vi "PumpValveHeater3.vi"() -> ()   [LabVIEW 2015]
uses:
  PumpValve.ctl
  <vilib>/DAQmx/read.llb/DAQmx Read (Analog 1D Wfm NChan 1Samp).vi
  <vilib>/DAQmx/write.llb/DAQmx Write (Digital 1D Bool NChan 1Samp 1Line).vi
  <vilib>/DAQmx/miscellaneous.llb/DAQmx Fill In Error Info.vi
  <vilib>/addons/control/pid/pid.llb/PID Advanced (DBL).vi
  <vilib>/addons/control/pid/NI_PID_pid.lvlib
panel:
  out "Pressure (mBar)":dbl format="%#_13g"
  out "Voltage Reading (Pressure)":dbl format="%#_13g"
  out "Pressure Chart Voltage":waveform(dbl)(graph)
  out "Voltage Reading(Temp)":dbl format="%#_13g"
  out "Temperature (Celcius)":dbl format="%#_13g"
  out "Temp(C)":dbl(slide) scale=-10.0..100.0
  out "Temp Chart":waveform(dbl)(graph)
  out "Duty Cycle from Control Value":dbl
  out "Control Value Pressure":dbl
  out "Heater On/off":bool
  out "Control Value (Temp Sensor)":dbl(knob) scale=0.0..100.0
  in  "PID gains Temp":T1={"proportional gain (Kc)"=1.0, "integral time (Ti, min)"=0.01, "derivative time (Td, min)"=0.0} {"derivative time (Td, min)" format="%.3f"; "integral time (Ti, min)" format="%.3f"; "proportional gain (Kc)" format="%.3f"}
  in  "Temp Setting":dbl
  in  "Maintain Temp":bool
  in  "Stop Maintaining Pressure":bool
  in  "PID gains":T1={"proportional gain (Kc)"=1.0, "integral time (Ti, min)"=0.01, "derivative time (Td, min)"=0.0} {"derivative time (Td, min)" format="%.3f"; "integral time (Ti, min)" format="%.3f"; "proportional gain (Kc)" format="%.3f"}
  out "Control Value (Pressure Sensor)":dbl(knob) scale=-10.0..10.0
  in  "Pressure Setting (mBar)":dbl
  in  "Maintain pressure":bool
  in  "On/Off Temp":bool
  in  "Manual Mode Temp":bool
  in  "Duty cycle % (0-100)":dbl=50.0
  in  "Steps in a cycle":i32=256
  in  "Cycle time (s)":dbl=5.0
  in  "On/Off (Pump)":bool
  in  "Open/Close (Blue)":bool
  in  "Open/Close (Green)":bool
  in  "Manual Mode Pump/Valve":bool
  out "Invalid fill%":bool
  out "Tank":u32(slide) scale=0.0..100.0
  in  "Drain %":u32
  in  "Fill %":u32
  in  "Drain":bool
  in  "Stop Program":bool
  in  "Fill":bool
  # "Temp only adjusts up (do nothing to cool?)"
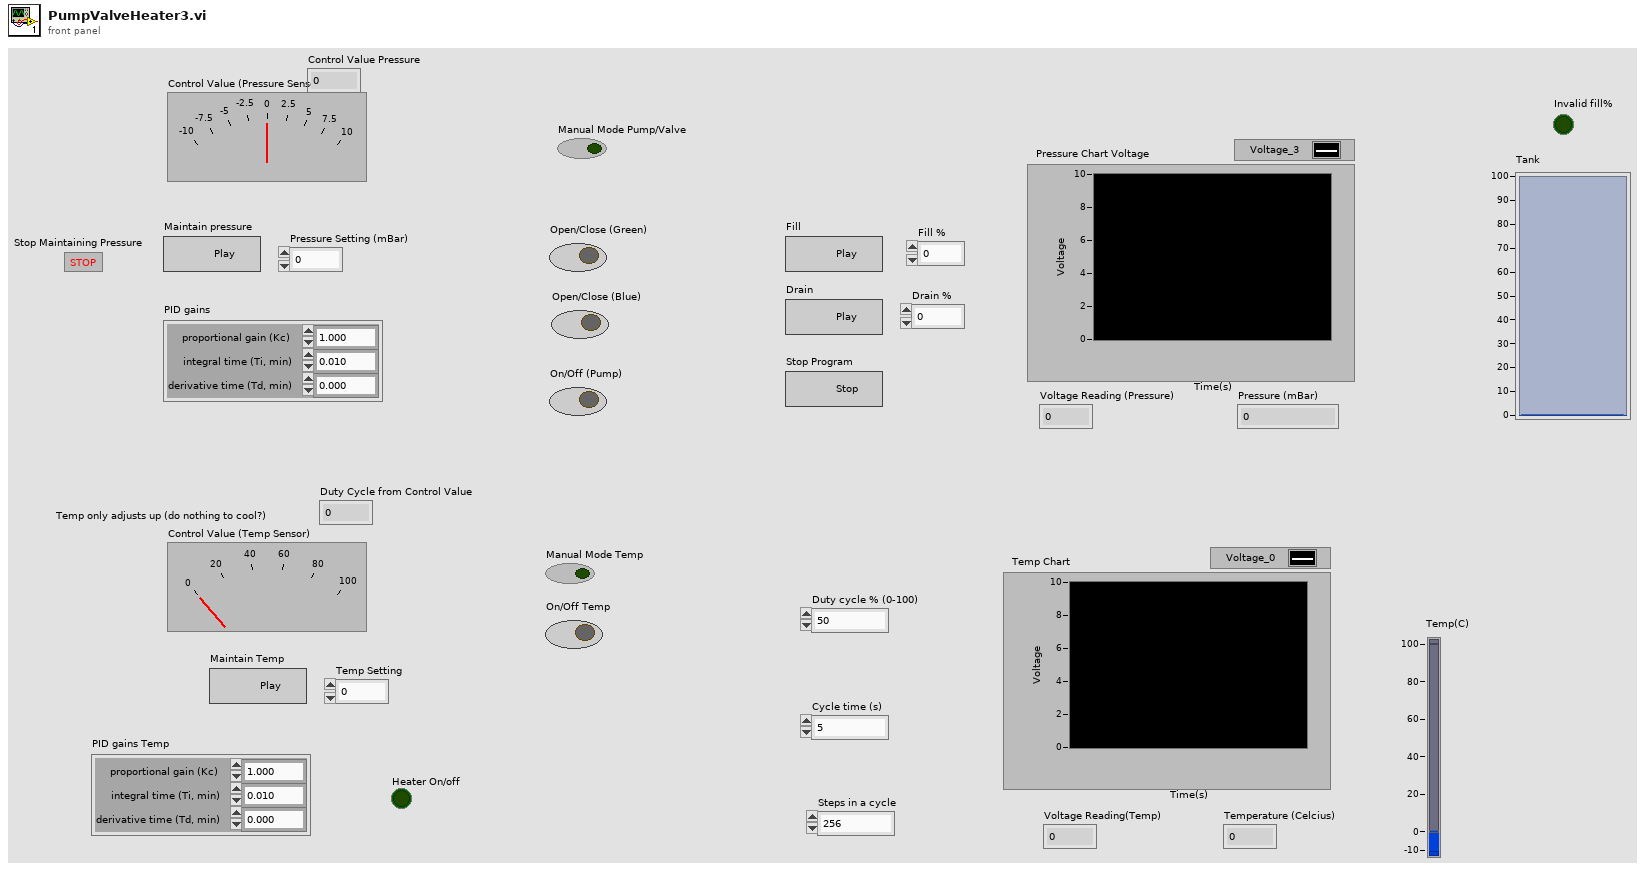
[diagram p1: front panel]
types:
  T1 = cluster{"proportional gain (Kc)":dbl, "integral time (Ti, min)":dbl, "derivative time (Td, min)":dbl}
  T2 = typedef "PumpValve.ctl" = enum16{"PressureSetting", "ManualPressure", "ManualTemp", "Idle Temp", "Set Temp", "Initialize", "Idle", "Fill", "Drain", "Stop"}
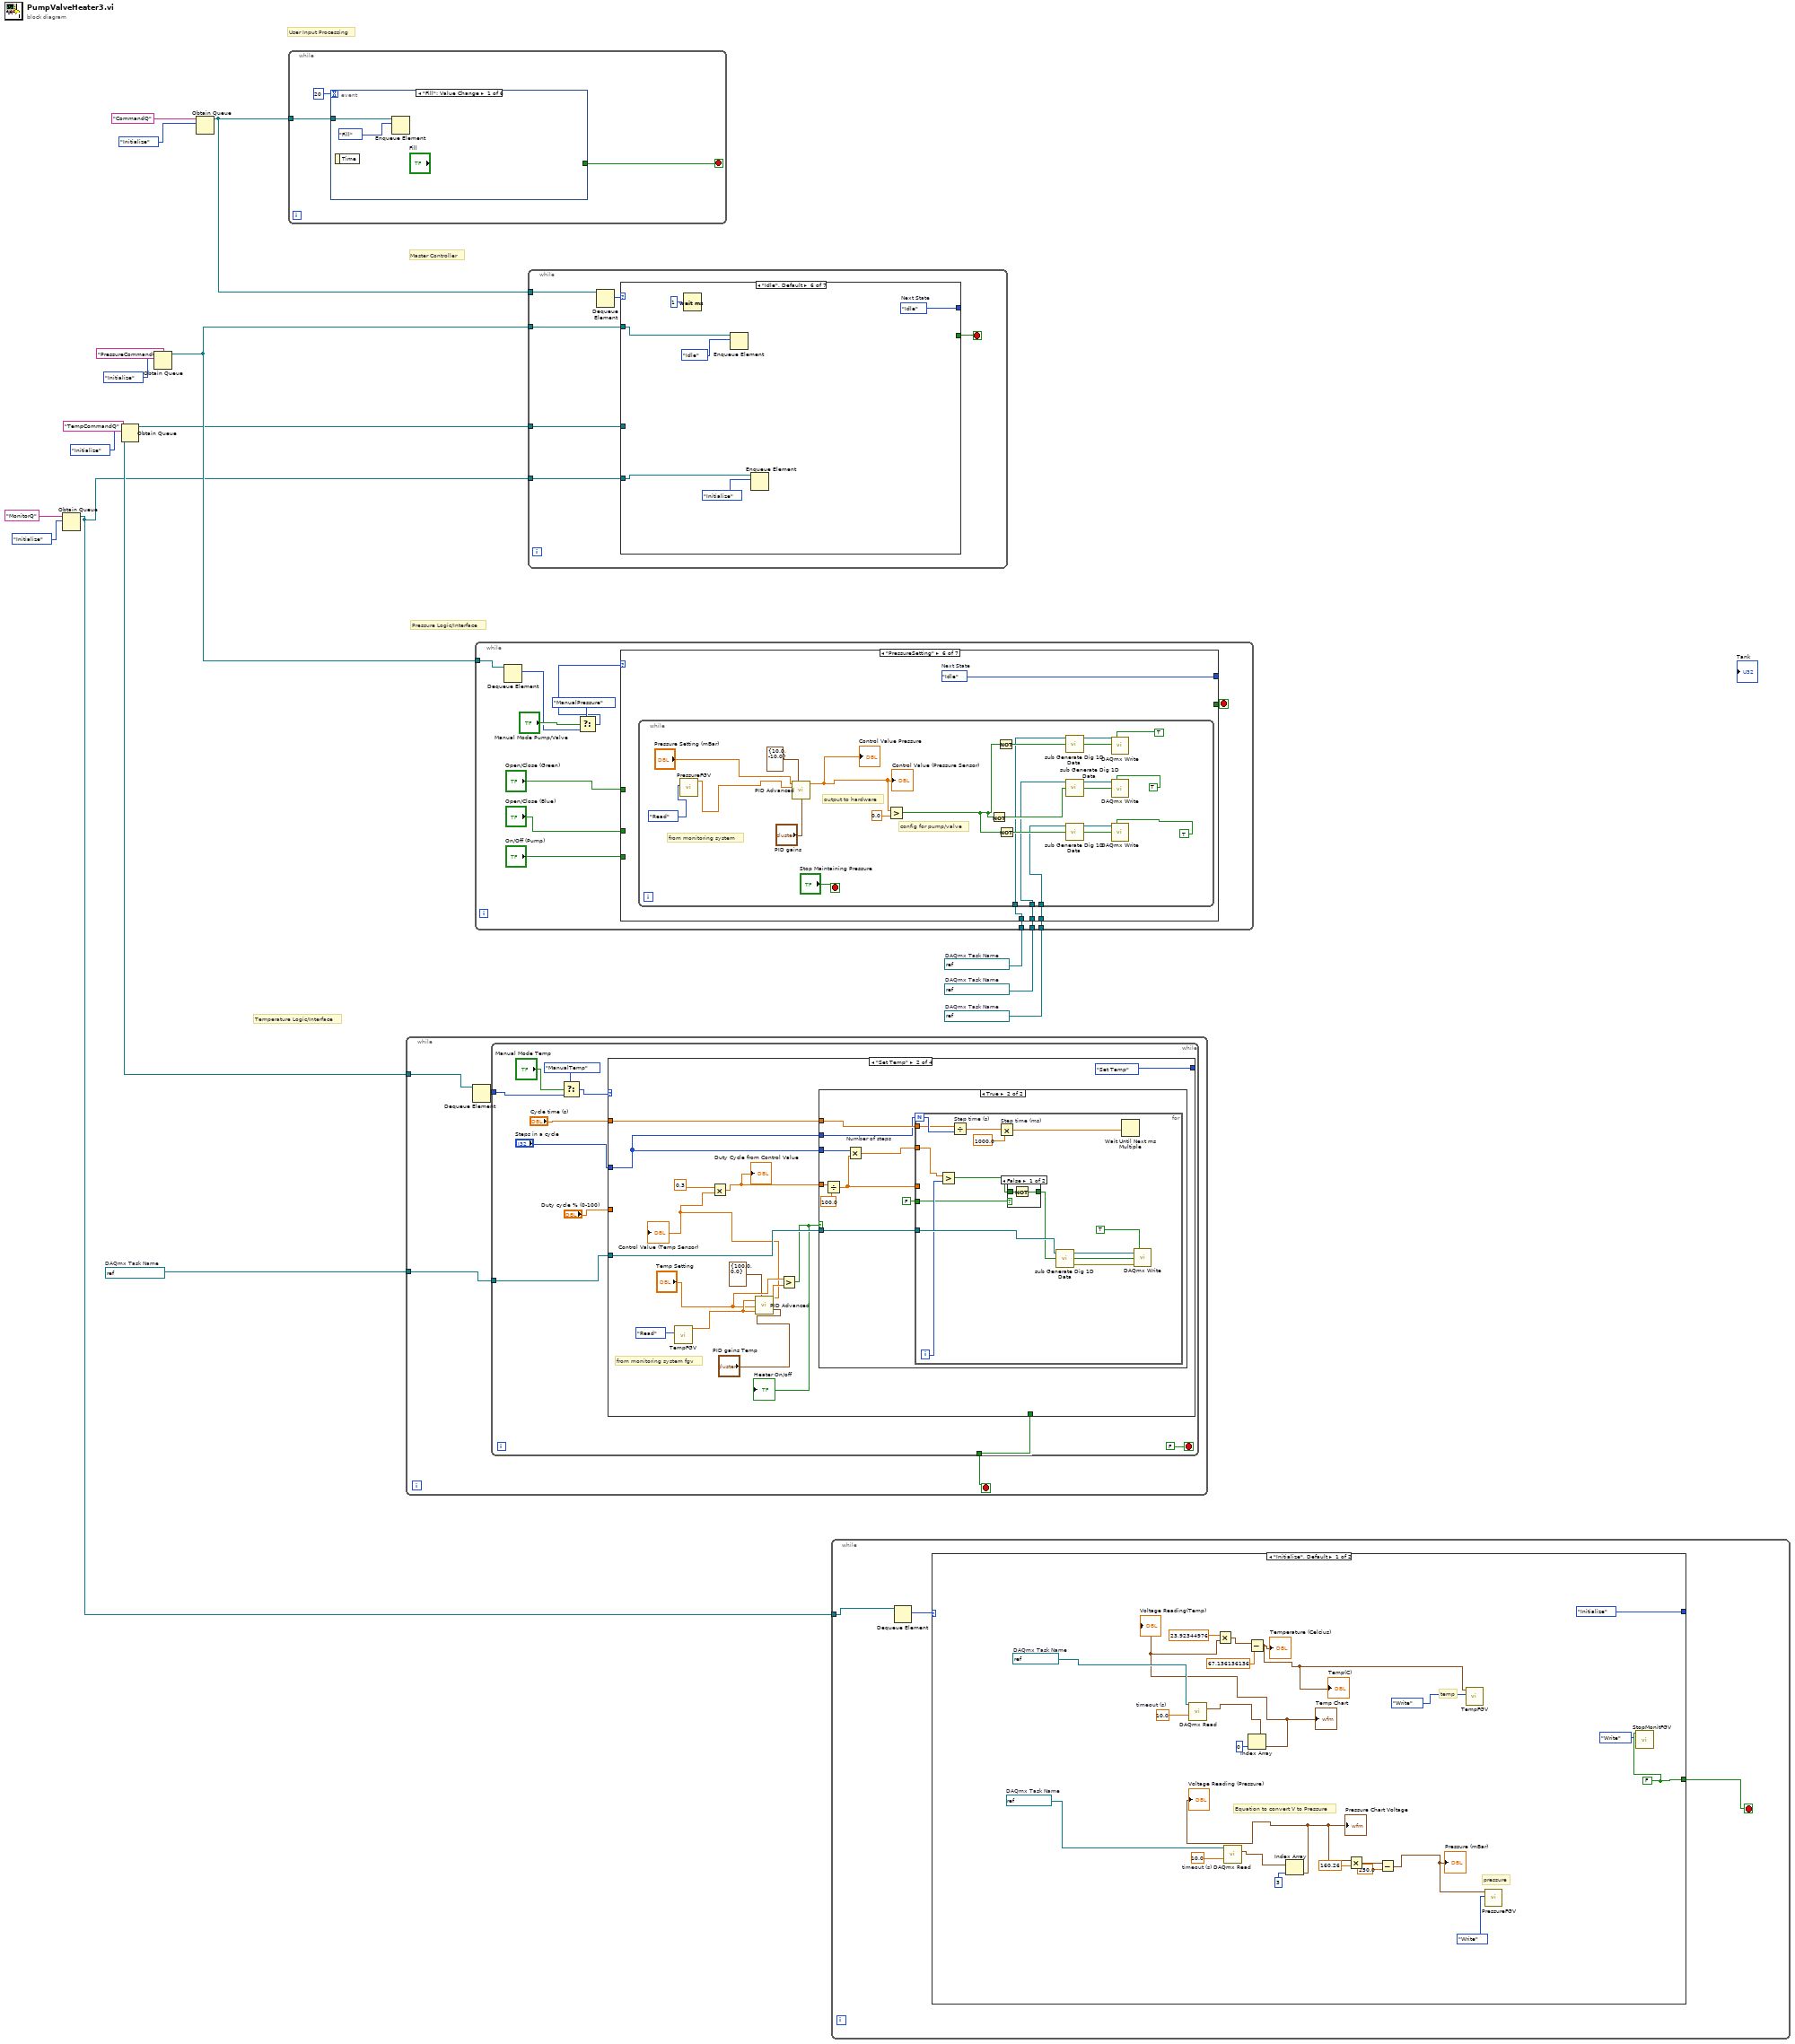
[diagram p0: block diagram]
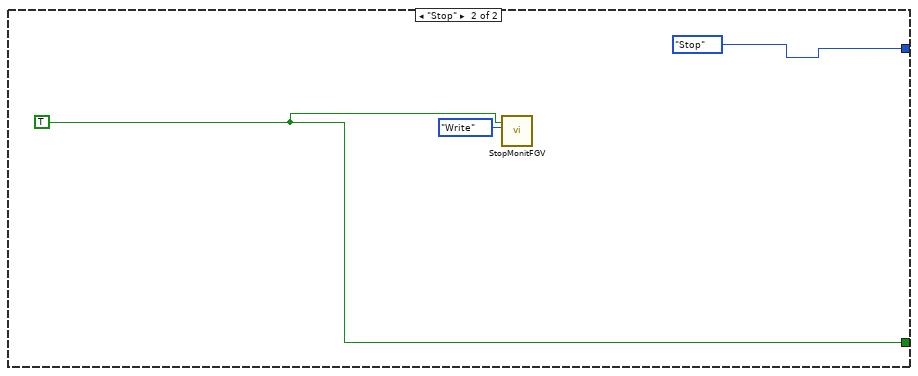
[diagram p2: hidden frame]
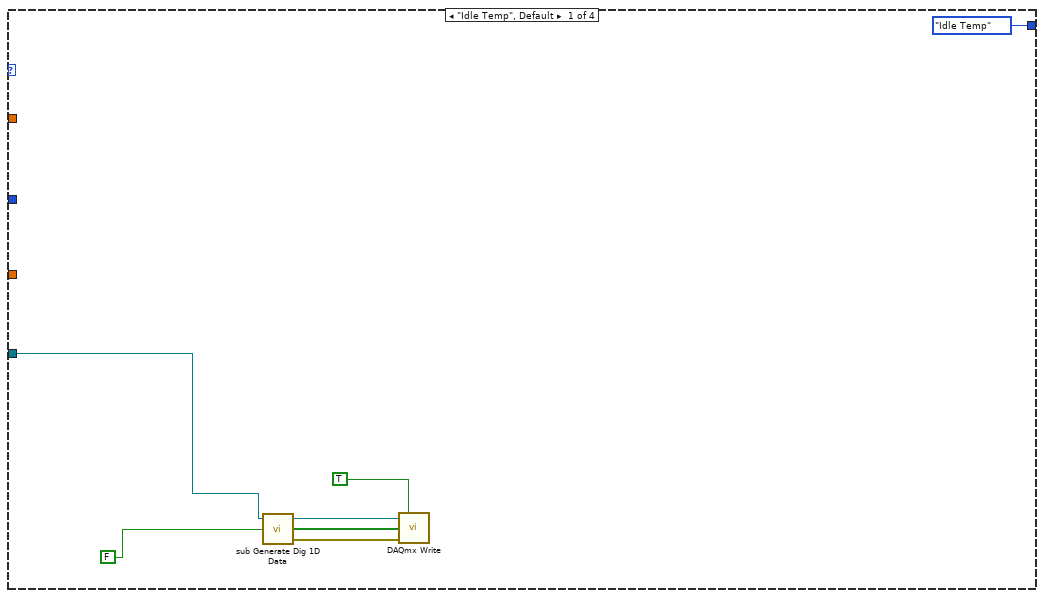
[diagram p3: hidden frame]
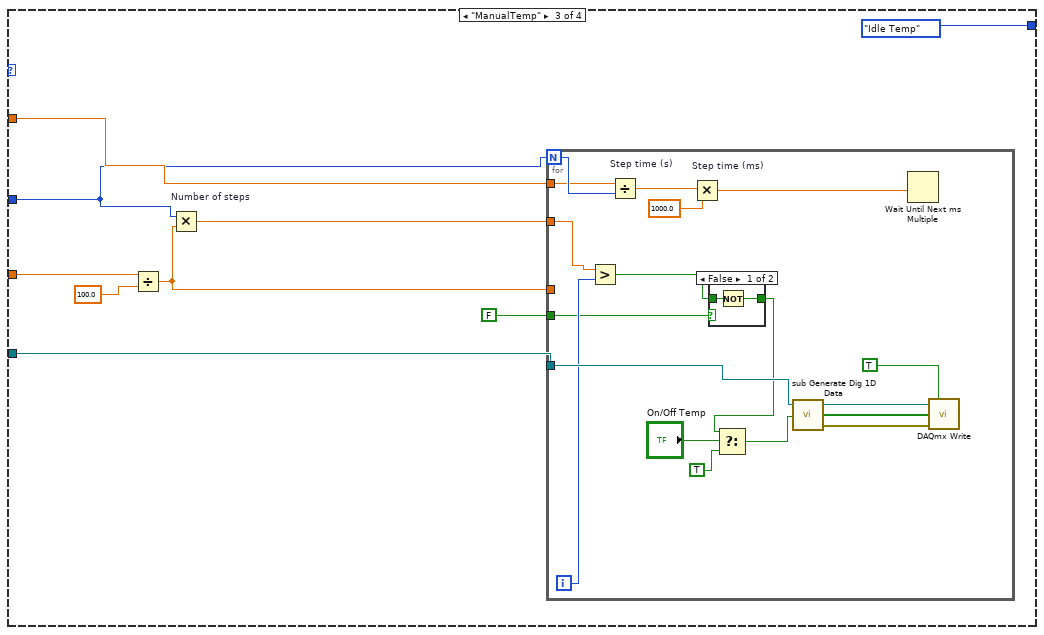
[diagram p6: hidden frame]
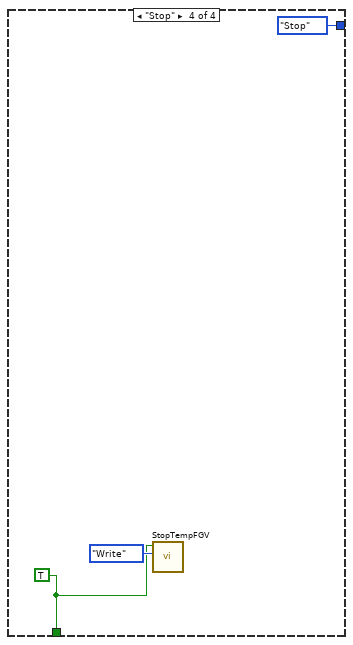
[diagram p8: hidden frame]
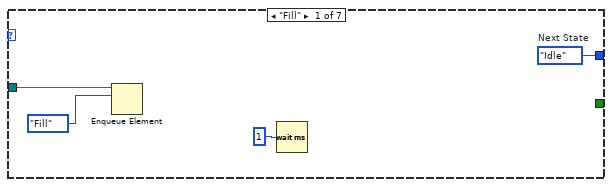
[diagram p9: hidden frame]
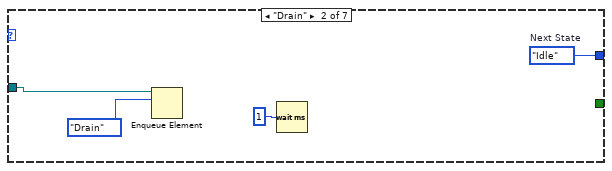
[diagram p10: hidden frame]
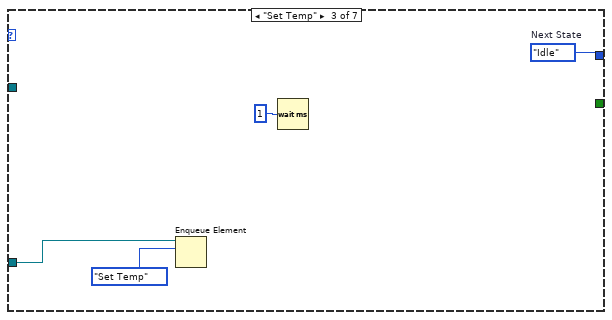
[diagram p11: hidden frame]
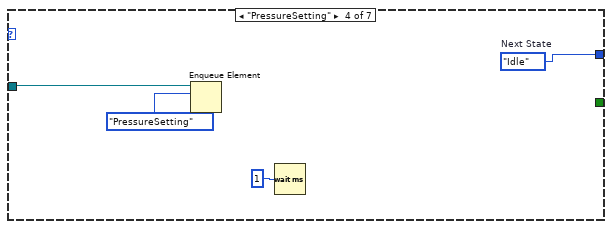
[diagram p12: hidden frame]
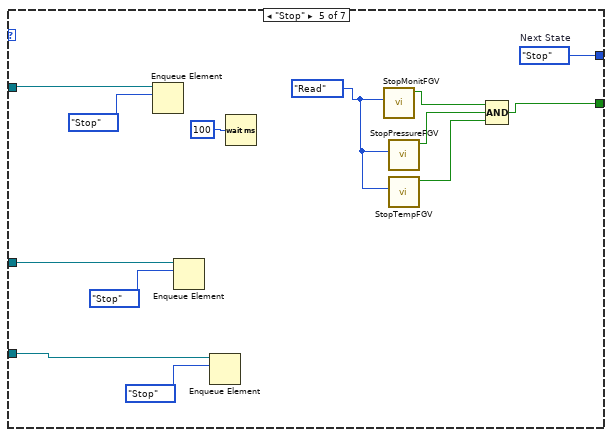
[diagram p13: hidden frame]
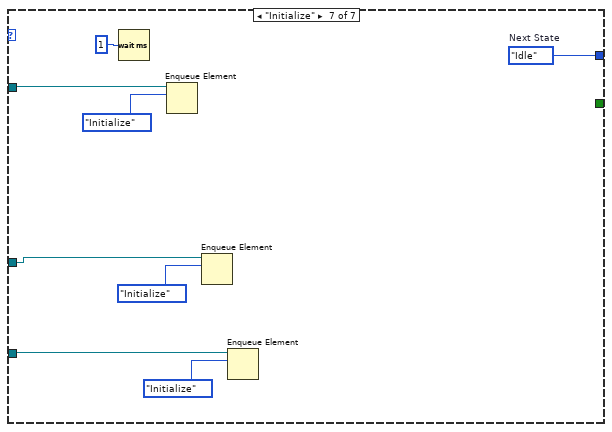
[diagram p14: hidden frame]
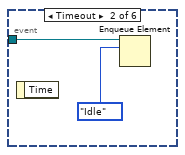
[diagram p15: hidden frame]
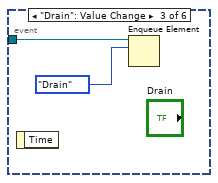
[diagram p16: hidden frame]
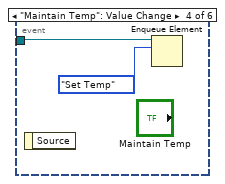
[diagram p17: hidden frame]
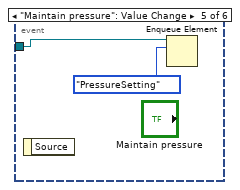
[diagram p18: hidden frame]
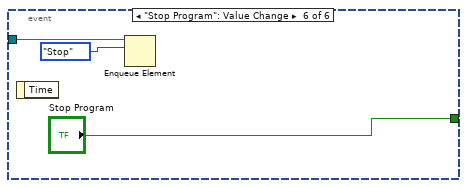
[diagram p19: hidden frame]
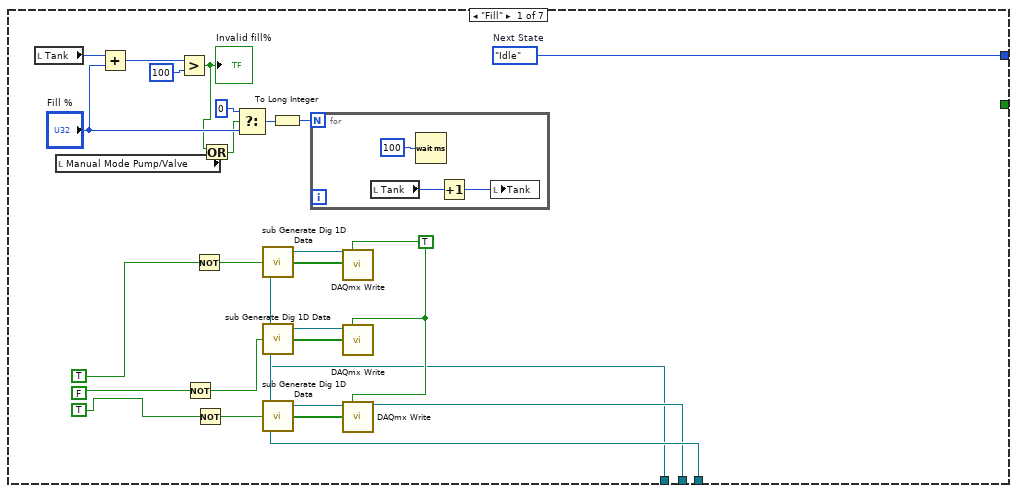
[diagram p20: hidden frame]
diagram:
  w7 = refnum<k21> "YellowdigOUT"  # DAQmx Task Name
  w12 = refnum<k21> "DigitalOutGreen"  # DAQmx Task Name
  w13 = refnum<k21> "DigitalOutGreen"  # DAQmx Task Name
  w14 = refnum<k21> "DigitalOutGreen"  # DAQmx Task Name
  # "Temperature Logic/Interface"
  # "Pressure Logic/Interface"
  # "Master Controller"
  # "User Input Processing"
  n1 = Obtain Queue(name (unnamed)="MonitorQ", element data type=PumpValve."Initialize" ("States")) -> (queue out=w1:refnum<queue>)  [unwired: 3 in, 2 out]
  n2 = Obtain Queue(name (unnamed)="TempCommandQ", element data type=PumpValve."Initialize" ("States")) -> (queue out=w4:refnum<queue>)  [unwired: 3 in, 2 out]
  n3 = Obtain Queue(name (unnamed)="PressureCommandQ", element data type=PumpValve."Initialize" ("States")) -> (queue out=w8:refnum<queue>)  [unwired: 3 in, 2 out]
  n4 = Obtain Queue(name (unnamed)="CommandQ", element data type=PumpValve."Initialize" ("States")) -> (queue out=w11:refnum<queue>)  [unwired: 3 in, 2 out]
  n5 = while {
    tunnel: w11 -> [w18]
    stop <- w17 stop-if-true
    n6 = event shown="[0] \"Fill\": Value Change" {
      selector: _ -> [_ _ _ _ _ _]
      dyn-events: _ -> [_ _ _ _ _ _]
      timeout: 20 -> [_ _ _ _ _ _]
      tunnel: w18 -> [w21 w23 w25 w26 w29 w32]
      tunnel: [_ _ _ _ _ "Stop Program"] -> w17
      event "Fill": Value Change {
        n7 = event-data() -> ()  [unwired: 1 in, 1 out]
        n8 = Enqueue Element(queue=w21, element=PumpValve."Fill" ("States")) -> ()  [unwired: 2 in, 3 out]
      }
      event Timeout {
        n9 = event-data() -> ()  [unwired: 1 in, 1 out]
        n10 = Enqueue Element(queue=w23, element=PumpValve."Idle" ("States")) -> ()  [unwired: 2 in, 3 out]
      }
      event "Drain": Value Change {
        n11 = event-data() -> ()  [unwired: 1 in, 1 out]
        n12 = Enqueue Element(queue=w25, element=PumpValve."Drain" ("States")) -> ()  [unwired: 2 in, 3 out]
      }
      event "Maintain Temp": Value Change {
        n13 = event-data() -> ()  [unwired: 1 in, 1 out]
        n14 = Enqueue Element(queue=w26, element=PumpValve."Set Temp" ("States")) -> ()  [unwired: 2 in, 3 out]
      }
      event "Maintain pressure": Value Change {
        n15 = event-data() -> ()  [unwired: 1 in, 1 out]
        n16 = Enqueue Element(queue=w29, element=PumpValve."PressureSetting" ("States")) -> ()  [unwired: 2 in, 3 out]
      }
      event "Stop Program": Value Change {
        n17 = event-data() -> ()  [unwired: 1 in, 1 out]
        n18 = Enqueue Element(queue=w32, element=PumpValve."Stop" ("States")) -> ()  [unwired: 2 in, 3 out]
      }
    }
  }
  n19 = while {
    tunnel: w7 -> [w36]
    tunnel: w4 -> [w35]
    stop <- w33 stop-if-true
    n20 = Dequeue Element(queue=w35) -> (element=w34:T2)  [unwired: 2 in, 3 out]
    n21 = while {
      tunnel: w36 -> [w46]
      tunnel: w34 -> [w45]
      tunnel: [w44] -> w33
      stop <- FALSE stop-if-true
      n22 = Select(t=PumpValve."ManualTemp", s="Manual Mode Temp", f=w45) -> (s? t:f=w40:T2)
      n23 = case shown="\"Set Temp\"" w40 {
        tunnel: w46 -> [w48 w66 w101 _]
        tunnel: [PumpValve."Idle Temp" ("States") PumpValve."Set Temp" ("States") PumpValve."Idle Temp" ("States") PumpValve."Stop" ("States")] -> _
        tunnel: "Cycle time (s)" -> [_ w64 w95 _]
        tunnel: "Steps in a cycle" -> [_ w63 w94 _]
        tunnel: "Duty cycle % (0-100)" -> [_ _ w93 _]
        tunnel: [_ _ _ w124] -> w44
        frame "Idle Temp", Default {
          n24 = call <vilib>:"sub Generate Dig 1D Data.vi"("initial value"=FALSE, "task in"=w48) -> ("error out"=w50:errorcluster, "Data"=w51:bool[], "task out"=w52:refnum<k21>)  [unwired: 1 in]
          n25 = call-poly <vilib>:"DAQmx Write.vi"("task/channels in"=w52, "auto start"=TRUE, "data"=w51, "error in"=w50) -> ()  [unwired: 9 in, 3 out]
        }
        frame "Set Temp" {
          # "from monitoring system fgv"
          n26 = call "TempFGV.vi"("Command"=enum16{"Write", "Read"}."Read") -> ("OUT"=w57:dbl)  [unwired: 10 in]
          n27 = call-poly <vilib>:"PID Advanced.vi"("setpoint"="Temp Setting", "output range"=cluster{"output high":dbl, "output low":dbl} {"output high"=100.0, "output low"=0.0}, "process variable"=w57, "PID gains"="PID gains Temp") -> ("output"=w55:dbl)  [unwired: 10 in, 1 out]
          "Control Value (Temp Sensor)" <- w55
          n28 = Multiply(x=0.3, y=w55) -> (x*y=w59:dbl)
          "Duty Cycle from Control Value" <- w59
          n29 = Greater?(x="Temp Setting", y=w57) -> (0:w62:bool)
          "Heater On/off" <- w62
          n30 = case shown="True" w62 {
            tunnel: w66 -> [_ w74]
            tunnel: w64 -> [_ w69]
            tunnel: w63 -> [_ w68]
            tunnel: w59 -> [_ w67]
            tunnel: w63 -> [_ _]
            frame False {
            }
            frame True {
              n31 = Divide(x=w67, y=100.0) -> (x/y=w72:dbl)
              n32 = Multiply "Number of steps"(x=w68, y=w72) -> (x*y=w71:dbl)
              n33 = for {
                N: w68 -> [w84]
                tunnel: w74 -> [w86]
                tunnel: w72 -> [_]
                tunnel: w69 -> [w83]
                tunnel: w71 -> [w79]
                tunnel: FALSE -> [w76]
                i -> [w78]
                n34 = Greater?(x=w79, y=w78) -> (0:w77:bool)
                n35 = Divide "Step time (s)"(x=w83, y=w84) -> (x/y=w82:dbl)
                n36 = Multiply "Step time (ms)"(x=w82, y=1000.0) -> (x*y=w80:dbl)
                n37 = case shown="False" w76 {
                  tunnel: [w90 w92] -> w85
                  tunnel: w77 -> [w91 w92]
                  frame False {
                    n38 = Not(x=w91) -> (.not. x?=w90:bool)
                  }
                  frame True {
                  }
                }
                n39 = call <vilib>:"sub Generate Dig 1D Data.vi"("initial value"=w85, "task in"=w86) -> ("error out"=w88:errorcluster, "Data"=w75:bool[], "task out"=w87:refnum<k21>)  [unwired: 1 in]
                n40 = Wait Until Next ms Multiple(millisecond multiple=w80) -> ()  [unwired: 1 out]
                n41 = call-poly <vilib>:"DAQmx Write.vi"("task/channels in"=w87, "auto start"=TRUE, "data"=w75, "error in"=w88) -> ()  [unwired: 9 in, 3 out]
              }
            }
          }
        }
        frame "ManualTemp" {
          n42 = Divide(x=w93, y=100.0) -> (x/y=w99:dbl)
          n43 = Multiply "Number of steps"(x=w94, y=w99) -> (x*y=w98:dbl)
          n44 = for {
            N: w94 -> [w114]
            tunnel: w101 -> [w115]
            tunnel: w99 -> [_]
            tunnel: w95 -> [w113]
            tunnel: w98 -> [w109]
            tunnel: FALSE -> [w106]
            i -> [w108]
            n45 = Greater?(x=w109, y=w108) -> (0:w107:bool)
            n46 = Divide "Step time (s)"(x=w113, y=w114) -> (x/y=w112:dbl)
            n47 = Multiply "Step time (ms)"(x=w112, y=1000.0) -> (x*y=w110:dbl)
            n48 = case shown="False" w106 {
              tunnel: [w120 w122] -> w104
              tunnel: w107 -> [w121 w122]
              frame False {
                n49 = Not(x=w121) -> (.not. x?=w120:bool)
              }
              frame True {
              }
            }
            n50 = Select(t=w104, s="On/Off Temp", f=TRUE) -> (s? t:f=w103:bool)
            n51 = call <vilib>:"sub Generate Dig 1D Data.vi"("initial value"=w103, "task in"=w115) -> ("error out"=w118:errorcluster, "Data"=w117:bool[], "task out"=w116:refnum<k21>)  [unwired: 1 in]
            n52 = Wait Until Next ms Multiple(millisecond multiple=w110) -> ()  [unwired: 1 out]
            n53 = call-poly <vilib>:"DAQmx Write.vi"("task/channels in"=w116, "auto start"=TRUE, "data"=w117, "error in"=w118) -> ()  [unwired: 9 in, 3 out]
          }
        }
        frame "Stop" {
          w124 = TRUE
          n54 = call "StopTempFGV.vi"("Command"=enum16{"Write", "Read"}."Write", "IN"=w124) -> ()  [unwired: 9 in, 1 out]
        }
      }
    }
  }
  n55 = while {
    tunnel: w8 -> [w137]
    tunnel: w14 -> [w133]
    tunnel: w13 -> [w134]
    tunnel: w12 -> [w135]
    stop <- w136 stop-if-true
    n56 = Dequeue Element(queue=w137) -> (element=w130:T2)  [unwired: 2 in, 3 out]
    n57 = Select(t=PumpValve."ManualPressure", s="Manual Mode Pump/Valve", f=w130) -> (s? t:f=w129:T2)
    n58 = case shown="\"PressureSetting\"" w129 {
      tunnel: [w164 w192 w214 w236 w256 w260 w306] -> _
      tunnel: [_ _ w197 _ _ _ _] -> w136
      tunnel: w135 -> [w146 w174 w204 w224 w244 w257 w295]
      tunnel: w134 -> [w145 w175 w205 w223 w243 w258 w296]
      tunnel: w133 -> [w144 w176 w206 w222 w242 w259 w297]
      tunnel: "Open/Close (Green)" -> [_ _ _ _ w239 _ _]
      tunnel: "Open/Close (Blue)" -> [_ _ _ _ w238 _ _]
      tunnel: "On/Off (Pump)" -> [_ _ _ _ w237 _ _]
      frame "Fill" {
        w153 = TRUE
        w164 = PumpValve."Idle"  # Next State
        n59 = local read "Tank"() -> (w163:u32)
        n60 = local read "Manual Mode Pump/Valve"() -> (w155:bool)
        n61 = Add(x=w163, y="Fill %") -> (x+y=w161:u32)
        n62 = Greater?(x=w161, y=u32 100) -> (0:w156:bool)
        "Invalid fill%" <- w156
        n63 = Not(x=FALSE) -> (.not. x?=w141:bool)
        n64 = Not(x=TRUE) -> (.not. x?=w142:bool)
        n65 = Not(x=TRUE) -> (.not. x?=w143:bool)
        n66 = Or(x=w156, y=w155) -> (x .or. y?=w154:bool)
        n67 = Select(t=u32 0, s=w154, f="Fill %") -> (s? t:f=w158:u32)
        n68 = call <vilib>:"sub Generate Dig 1D Data.vi"("initial value"=w142, "task in"=w144) -> ("Data"=w148:bool[], "task out"=w152:refnum<k21>)  [unwired: 1 in, 1 out]
        n69 = call <vilib>:"sub Generate Dig 1D Data.vi"("initial value"=w141, "task in"=w145) -> ("Data"=w149:bool[], "task out"=w151:refnum<k21>)  [unwired: 1 in, 1 out]
        n70 = call <vilib>:"sub Generate Dig 1D Data.vi"("initial value"=w143, "task in"=w146) -> ("Data"=w147:bool[], "task out"=w150:refnum<k21>)  [unwired: 1 in, 1 out]
        n71 = To Long Integer(number=w158) -> (32bit integer=w157:i32)
        n72 = for {
          N: w157 -> [_]
          n73 = local read "Tank"() -> (w167:u32)
          n74 = Wait (ms)(milliseconds to wait=u32 100 ("y")) -> ()  [unwired: 1 out]
          n75 = Increment(x=w167) -> (x+1=w166:u32)
          n76 = local write "Tank"(w166) -> ()
        }
        n77 = call-poly <vilib>:"DAQmx Write.vi"("task/channels in"=w152, "auto start"=w153, "data"=w148) -> ()  [unwired: 10 in, 3 out]
        n78 = call-poly <vilib>:"DAQmx Write.vi"("task/channels in"=w151, "auto start"=w153, "data"=w149) -> ()  [unwired: 10 in, 3 out]
        n79 = call-poly <vilib>:"DAQmx Write.vi"("task/channels in"=w150, "auto start"=w153, "data"=w147) -> ()  [unwired: 10 in, 3 out]
      }
      frame "Drain" {
        w177 = TRUE
        w192 = PumpValve."Idle"  # Next State
        n80 = local read "Tank"() -> (w189:u32)
        n81 = local read "Manual Mode Pump/Valve"() -> (w187:bool)
        n82 = Greater?(x="Drain %", y=w189) -> (0:w188:bool)
        n83 = Select(t=w189, s=w188, f="Drain %") -> (s? t:f=w191:u32)
        n84 = Not(x=FALSE) -> (.not. x?=w172:bool)
        n85 = Not(x=TRUE) -> (.not. x?=w171:bool)
        n86 = Not(x=TRUE) -> (.not. x?=w173:bool)
        n87 = To Long Integer(number=w191) -> (32bit integer=w184:i32)
        n88 = Select(t=0, s=w187, f=w184) -> (s? t:f=w185:i32)
        n89 = for {
          N: w185 -> [_]
          n90 = local read "Tank"() -> (w194:u32)
          n91 = Wait (ms)(milliseconds to wait=u32 100) -> ()  [unwired: 1 out]
          n92 = Decrement(x=w194) -> (x-1=w195:u32)
          n93 = local write "Tank"(w195) -> ()
        }
        n94 = call <vilib>:"sub Generate Dig 1D Data.vi"("initial value"=w172, "task in"=w176) -> ("Data"=w182:bool[], "task out"=w178:refnum<k21>)  [unwired: 1 in, 1 out]
        n95 = call <vilib>:"sub Generate Dig 1D Data.vi"("initial value"=w171, "task in"=w175) -> ("Data"=w181:bool[], "task out"=w179:refnum<k21>)  [unwired: 1 in, 1 out]
        n96 = call <vilib>:"sub Generate Dig 1D Data.vi"("initial value"=w173, "task in"=w174) -> ("Data"=w183:bool[], "task out"=w180:refnum<k21>)  [unwired: 1 in, 1 out]
        n97 = call-poly <vilib>:"DAQmx Write.vi"("task/channels in"=w178, "auto start"=w177, "data"=w182) -> ()  [unwired: 10 in, 3 out]
        n98 = call-poly <vilib>:"DAQmx Write.vi"("task/channels in"=w179, "auto start"=w177, "data"=w181) -> ()  [unwired: 10 in, 3 out]
        n99 = call-poly <vilib>:"DAQmx Write.vi"("task/channels in"=w180, "auto start"=w177, "data"=w183) -> ()  [unwired: 10 in, 3 out]
      }
      frame "Stop" {
        w213 = TRUE
        w197 = TRUE  # Off
        w214 = PumpValve."Stop"  # Next State
        n100 = Not(x=FALSE) -> (.not. x?=w201:bool)
        n101 = Not(x=FALSE) -> (.not. x?=w202:bool)
        n102 = Not(x=FALSE) -> (.not. x?=w203:bool)
        n103 = call <vilib>:"sub Generate Dig 1D Data.vi"("initial value"=w202, "task in"=w206) -> ("Data"=w208:bool[], "task out"=w212:refnum<k21>)  [unwired: 1 in, 1 out]
        n104 = call <vilib>:"sub Generate Dig 1D Data.vi"("initial value"=w201, "task in"=w205) -> ("Data"=w209:bool[], "task out"=w211:refnum<k21>)  [unwired: 1 in, 1 out]
        n105 = call <vilib>:"sub Generate Dig 1D Data.vi"("initial value"=w203, "task in"=w204) -> ("Data"=w207:bool[], "task out"=w210:refnum<k21>)  [unwired: 1 in, 1 out]
        n106 = call-poly <vilib>:"DAQmx Write.vi"("task/channels in"=w212, "auto start"=w213, "data"=w208) -> ()  [unwired: 10 in, 3 out]
        n107 = call-poly <vilib>:"DAQmx Write.vi"("task/channels in"=w211, "auto start"=w213, "data"=w209) -> ()  [unwired: 10 in, 3 out]
        n108 = call-poly <vilib>:"DAQmx Write.vi"("task/channels in"=w210, "auto start"=w213, "data"=w207) -> ()  [unwired: 10 in, 3 out]
        n109 = call "StopPressureFGV.vi"("Command"=enum16{"Write", "Read"}."Write", "IN"=w197) -> ()  [unwired: 9 in, 1 out]
      }
      frame "Idle", Default {
        w236 = PumpValve."Idle"  # Next State
        n110 = Wait (ms)(milliseconds to wait=u32 10) -> ()  [unwired: 1 out]
        n111 = Not(x=FALSE) -> (.not. x?=w220:bool)
        n112 = Not(x=FALSE) -> (.not. x?=w221:bool)
        n113 = Not(x=FALSE) -> (.not. x?=w227:bool)
        n114 = call <vilib>:"sub Generate Dig 1D Data.vi"("initial value"=w221, "task in"=w222) -> ("Data"=w229:bool[], "task out"=w233:refnum<k21>)  [unwired: 1 in, 1 out]
        n115 = call <vilib>:"sub Generate Dig 1D Data.vi"("initial value"=w220, "task in"=w223) -> ("Data"=w230:bool[], "task out"=w232:refnum<k21>)  [unwired: 1 in, 1 out]
        n116 = call <vilib>:"sub Generate Dig 1D Data.vi"("initial value"=w227, "task in"=w224) -> ("Data"=w228:bool[], "task out"=w231:refnum<k21>)  [unwired: 1 in, 1 out]
        n117 = call-poly <vilib>:"DAQmx Write.vi"("task/channels in"=w233, "auto start"=TRUE, "data"=w229) -> ()  [unwired: 10 in, 3 out]
        n118 = call-poly <vilib>:"DAQmx Write.vi"("task/channels in"=w232, "auto start"=TRUE, "data"=w230) -> ()  [unwired: 10 in, 3 out]
        n119 = call-poly <vilib>:"DAQmx Write.vi"("task/channels in"=w231, "auto start"=TRUE, "data"=w228) -> ()  [unwired: 10 in, 3 out]
        n120 = call "StopPressureFGV.vi"("Command"=enum16{"Write", "Read"}."Write", "IN"=FALSE) -> ()  [unwired: 9 in, 1 out]
      }
      frame "ManualPressure" {
        w256 = PumpValve."Idle"  # Next State
        n121 = Wait (ms)(milliseconds to wait=u32 10) -> ()  [unwired: 1 out]
        n122 = Not(x=w238) -> (.not. x?=w240:bool)
        n123 = Not(x=w239) -> (.not. x?=w241:bool)
        n124 = Not(x=w237) -> (.not. x?=w247:bool)
        n125 = call <vilib>:"sub Generate Dig 1D Data.vi"("initial value"=w241, "task in"=w242) -> ("Data"=w249:bool[], "task out"=w253:refnum<k21>)  [unwired: 1 in, 1 out]
        n126 = call <vilib>:"sub Generate Dig 1D Data.vi"("initial value"=w240, "task in"=w243) -> ("Data"=w250:bool[], "task out"=w252:refnum<k21>)  [unwired: 1 in, 1 out]
        n127 = call <vilib>:"sub Generate Dig 1D Data.vi"("initial value"=w247, "task in"=w244) -> ("Data"=w248:bool[], "task out"=w251:refnum<k21>)  [unwired: 1 in, 1 out]
        n128 = call-poly <vilib>:"DAQmx Write.vi"("task/channels in"=w253, "auto start"=TRUE, "data"=w249) -> ()  [unwired: 10 in, 3 out]
        n129 = call-poly <vilib>:"DAQmx Write.vi"("task/channels in"=w252, "auto start"=TRUE, "data"=w250) -> ()  [unwired: 10 in, 3 out]
        n130 = call-poly <vilib>:"DAQmx Write.vi"("task/channels in"=w251, "auto start"=TRUE, "data"=w248) -> ()  [unwired: 10 in, 3 out]
      }
      frame "PressureSetting" {
        w260 = PumpValve."Idle"  # Next State
        n131 = while {
          tunnel: w259 -> [w264]
          tunnel: w258 -> [w263]
          tunnel: w257 -> [w262]
          stop <- "Stop Maintaining Pressure" stop-if-true
          # "config for pump/valve"
          # "from monitoring system"
          # "output to hardware"
          n132 = call "PressureFGV.vi"("Command"=enum16{"Write", "Read"}."Read") -> ("OUT"=w281:dbl)  [unwired: 10 in]
          n133 = call-poly <vilib>:"PID Advanced.vi"("setpoint"="Pressure Setting (mBar)", "output range"=cluster{"output high":dbl, "output low":dbl} {"output high"=10.0, "output low"=-10.0}, "process variable"=w281, "PID gains"="PID gains") -> ("output"=w278:dbl)  [unwired: 10 in, 1 out]
          "Control Value (Pressure Sensor)" <- w278
          "Control Value Pressure" <- w278
          n134 = Greater?(x=w278, y=0.0) -> (0:w261:bool)
          n135 = Not(x=w261) -> (.not. x?=w265:bool)
          n136 = Not(x=w261) -> (.not. x?=w266:bool)
          n137 = Not(x=w261) -> (.not. x?=w269:bool)
          n138 = call <vilib>:"sub Generate Dig 1D Data.vi"("initial value"=w266, "task in"=w264) -> ("Data"=w271:bool[], "task out"=w275:refnum<k21>)  [unwired: 1 in, 1 out]
          n139 = call <vilib>:"sub Generate Dig 1D Data.vi"("initial value"=w265, "task in"=w263) -> ("Data"=w272:bool[], "task out"=w274:refnum<k21>)  [unwired: 1 in, 1 out]
          n140 = call <vilib>:"sub Generate Dig 1D Data.vi"("initial value"=w269, "task in"=w262) -> ("Data"=w270:bool[], "task out"=w273:refnum<k21>)  [unwired: 1 in, 1 out]
          n141 = call-poly <vilib>:"DAQmx Write.vi"("task/channels in"=w275, "auto start"=TRUE, "data"=w271) -> ()  [unwired: 10 in, 3 out]
          n142 = call-poly <vilib>:"DAQmx Write.vi"("task/channels in"=w274, "auto start"=TRUE, "data"=w272) -> ()  [unwired: 10 in, 3 out]
          n143 = call-poly <vilib>:"DAQmx Write.vi"("task/channels in"=w273, "auto start"=TRUE, "data"=w270) -> ()  [unwired: 10 in, 3 out]
        }
      }
      frame "Initialize" {
        w306 = PumpValve."Idle"  # Next State
        n144 = Wait (ms)(milliseconds to wait=u32 1) -> ()  [unwired: 1 out]
        n145 = Not(x=FALSE) -> (.not. x?=w291:bool)
        n146 = Not(x=FALSE) -> (.not. x?=w290:bool)
        n147 = Not(x=FALSE) -> (.not. x?=w294:bool)
        n148 = call <vilib>:"sub Generate Dig 1D Data.vi"("initial value"=w291, "task in"=w297) -> ("Data"=w299:bool[], "task out"=w303:refnum<k21>)  [unwired: 1 in, 1 out]
        n149 = call <vilib>:"sub Generate Dig 1D Data.vi"("initial value"=w290, "task in"=w296) -> ("Data"=w300:bool[], "task out"=w302:refnum<k21>)  [unwired: 1 in, 1 out]
        n150 = call <vilib>:"sub Generate Dig 1D Data.vi"("initial value"=w294, "task in"=w295) -> ("Data"=w298:bool[], "task out"=w301:refnum<k21>)  [unwired: 1 in, 1 out]
        n151 = call-poly <vilib>:"DAQmx Write.vi"("task/channels in"=w303, "auto start"=TRUE, "data"=w299) -> ()  [unwired: 10 in, 3 out]
        n152 = call-poly <vilib>:"DAQmx Write.vi"("task/channels in"=w302, "auto start"=TRUE, "data"=w300) -> ()  [unwired: 10 in, 3 out]
        n153 = call-poly <vilib>:"DAQmx Write.vi"("task/channels in"=w301, "auto start"=TRUE, "data"=w298) -> ()  [unwired: 10 in, 3 out]
        n154 = call "StopPressureFGV.vi"("Command"=enum16{"Write", "Read"}."Write", "IN"=FALSE) -> ()  [unwired: 9 in, 1 out]
      }
    }
  }
  n155 = while {
    tunnel: w11 -> [w311]
    tunnel: w8 -> [w310]
    tunnel: w4 -> [w308]
    tunnel: w1 -> [w307]
    stop <- w309 stop-if-true
    n156 = Dequeue Element(queue=w311) -> (element=w312:T2)  [unwired: 2 in, 3 out]
    n157 = case shown="\"Idle\", Default" w312 {
      tunnel: [w316 w320 w322 w326 w341 w347 w355] -> _
      tunnel: w310 -> [w313 w317 _ w325 w338 w344 w352]
      tunnel: [_ _ _ _ w333 _ _] -> w309
      tunnel: w308 -> [_ _ w321 _ w336 _ w349]
      tunnel: w307 -> [_ _ _ _ w334 w342 w348]
      frame "Fill" {
        w316 = PumpValve."Idle"  # Next State
        n158 = Enqueue Element(queue=w313, element=PumpValve."Fill" ("States")) -> ()  [unwired: 2 in, 3 out]
        n159 = Wait (ms)(milliseconds to wait=u32 1) -> ()  [unwired: 1 out]
      }
      frame "Drain" {
        w320 = PumpValve."Idle"  # Next State
        n160 = Enqueue Element(queue=w317, element=PumpValve."Drain" ("States")) -> ()  [unwired: 2 in, 3 out]
        n161 = Wait (ms)(milliseconds to wait=u32 1) -> ()  [unwired: 1 out]
      }
      frame "Set Temp" {
        w322 = PumpValve."Idle"  # Next State
        n162 = Enqueue Element(queue=w321, element=PumpValve."Set Temp" ("States")) -> ()  [unwired: 2 in, 3 out]
        n163 = Wait (ms)(milliseconds to wait=u32 1) -> ()  [unwired: 1 out]
      }
      frame "PressureSetting" {
        w326 = PumpValve."Idle"  # Next State
        n164 = Enqueue Element(queue=w325, element=PumpValve."PressureSetting" ("States")) -> ()  [unwired: 2 in, 3 out]
        n165 = Wait (ms)(milliseconds to wait=u32 1) -> ()  [unwired: 1 out]
      }
      frame "Stop" {
        w332 = enum16{"Write", "Read"}."Read" ("Command")
        w341 = PumpValve."Stop"  # Next State
        n166 = Enqueue Element(queue=w338, element=PumpValve."Stop" ("States")) -> ()  [unwired: 2 in, 3 out]
        n167 = Enqueue Element(queue=w336, element=PumpValve."Stop" ("States")) -> ()  [unwired: 2 in, 3 out]
        n168 = Enqueue Element(queue=w334, element=PumpValve."Stop" ("States")) -> ()  [unwired: 2 in, 3 out]
        n169 = Wait (ms)(milliseconds to wait=u32 100) -> ()  [unwired: 1 out]
        n170 = call "StopMonitFGV.vi"("Command"=w332) -> ("OUT"=w331:bool)  [unwired: 10 in]
        n171 = call "StopPressureFGV.vi"("Command"=w332) -> ("OUT"=w330:bool)  [unwired: 10 in]
        n172 = call "StopTempFGV.vi"("Command"=w332) -> ("OUT"=w329:bool)  [unwired: 10 in]
        n173 = Compound Arithmetic op=AND(w331, w330, w329) -> (w333:bool)
      }
      frame "Idle", Default {
        w347 = PumpValve."Idle"  # Next State
        n174 = Wait (ms)(milliseconds to wait=u32 1) -> ()  [unwired: 1 out]
        n175 = Enqueue Element(queue=w344, element=PumpValve."Idle" ("States")) -> ()  [unwired: 2 in, 3 out]
        n176 = Enqueue Element(queue=w342, element=PumpValve."Initialize" ("States")) -> ()  [unwired: 2 in, 3 out]
      }
      frame "Initialize" {
        w355 = PumpValve."Idle"  # Next State
        n177 = Wait (ms)(milliseconds to wait=u32 1) -> ()  [unwired: 1 out]
        n178 = Enqueue Element(queue=w352, element=PumpValve."Initialize" ("States")) -> ()  [unwired: 2 in, 3 out]
        n179 = Enqueue Element(queue=w349, element=PumpValve."Initialize" ("States")) -> ()  [unwired: 2 in, 3 out]
        n180 = Enqueue Element(queue=w348, element=PumpValve."Initialize" ("States")) -> ()  [unwired: 2 in, 3 out]
      }
    }
  }
  n181 = while {
    tunnel: w1 -> [w358]
    stop <- w356 stop-if-true
    n182 = Dequeue Element(queue=w358) -> (element=w357:T2)  [unwired: 2 in, 3 out]
    n183 = case shown="\"Initialize\", Default" w357 {
      tunnel: [w379 w383] -> w356
      tunnel: [PumpValve."Initialize" ("States") PumpValve."Stop" ("States")] -> _
      frame "Initialize", Default {
        w371 = 10.0  # timeout (s)
        w377 = 10.0  # timeout (s)
        w380 = refnum<k21> "AllAnalog"  # DAQmx Task Name
        w381 = refnum<k21> "AllAnalog"  # DAQmx Task Name
        w379 = FALSE
        # "Equation to convert V to Pressure"
        # "pressure"
        # "temp"
        n184 = call-poly <vilib>:"DAQmx Read.vi"("task/channels in"=w381, "timeout"=w377) -> ("data"=w368:waveform(dbl)[])  [unwired: 11 in, 2 out]
        n185 = call-poly <vilib>:"DAQmx Read.vi"("task/channels in"=w380, "timeout"=w371) -> ("data"=w365:waveform(dbl)[])  [unwired: 11 in, 2 out]
        n186 = Index Array(array=w368, index=0) -> (element=w367:waveform(dbl))
        "Voltage Reading(Temp)" <- w367
        "Temp Chart" <- w367
        n187 = Multiply(x=23.92344976, y=w367) -> (x*y=w375:waveform(dbl))
        n188 = Subtract(x=w375, y=67.136136136) -> (x-y=w372:waveform(dbl))
        "Temperature (Celcius)" <- w372
        "Temp(C)" <- w372
        n189 = Index Array(array=w365, index=3) -> (element=w364:waveform(dbl))
        "Pressure Chart Voltage" <- w364
        "Voltage Reading (Pressure)" <- w364
        n190 = Multiply(x=w364, y=160.26) -> (x*y=w362:waveform(dbl))
        n191 = Subtract(x=w362, y=250.0) -> (x-y=w360:waveform(dbl))
        "Pressure (mBar)" <- w360
        n192 = call "TempFGV.vi"("Command"=enum16{"Write", "Read"}."Write", "IN"=w372) -> ()  [unwired: 9 in, 1 out]
        n193 = call "PressureFGV.vi"("Command"=enum16{"Write", "Read"}."Write", "IN"=w360) -> ()  [unwired: 9 in, 1 out]
        n194 = call "StopMonitFGV.vi"("Command"=enum16{"Write", "Read"}."Write", "IN"=w379) -> ()  [unwired: 9 in, 1 out]
      }
      frame "Stop" {
        w383 = TRUE
        n195 = call "StopMonitFGV.vi"("Command"=enum16{"Write", "Read"}."Write", "IN"=w383) -> ()  [unwired: 9 in, 1 out]
      }
    }
  }
